vi "reverse image.vi"(0 "output array in":dbl[][](array[numeric]), 1 "reverse h":bool, 2 "reverse v":bool) -> (3 "output array out":dbl[][](array[numeric]))   [LabVIEW 2018]
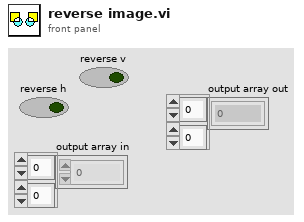
[diagram p1: front panel]
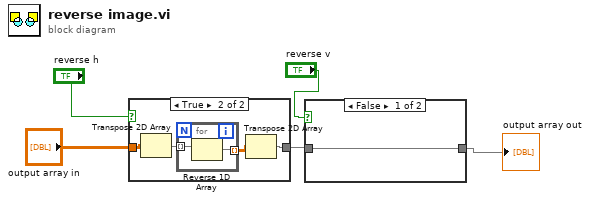
[diagram p0: block diagram]
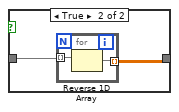
[diagram p2: hidden frame]
diagram:
  n1 = case shown="True" "reverse h" {
    tunnel: "output array in" -> [w6 w10]
    tunnel: [w6 w7] -> w3
    frame False {
    }
    frame True {
      n2 = Transpose 2D Array(2D array=w10) -> (transposed array=w9:dbl[][])
      n3 = for {
        tunnel: w9 -> [w12] mode=indexing
        tunnel: [w11] -> w8 mode=indexing
        n4 = Reverse 1D Array(array=w12) -> (reversed array=w11:dbl[])
      }
      n5 = Transpose 2D Array(2D array=w8) -> (transposed array=w7:dbl[][])
    }
  }
  n6 = case shown="False" "reverse v" {
    tunnel: w3 -> [w13 w15]
    tunnel: [w13 w14] -> w1
    frame False {
    }
    frame True {
      n7 = for {
        tunnel: w15 -> [w17] mode=indexing
        tunnel: [w16] -> w14 mode=indexing
        n8 = Reverse 1D Array(array=w17) -> (reversed array=w16:dbl[])
      }
    }
  }
  "output array out" <- w1
